vi "Database.GetProductComponentTable2.vi"(7 "ConnectionString":string, 10 "Component_SerialNo":string, 11 "Component_WabcoNo":string) -> (1 "Prod found":bool)   [LabVIEW 2016]
uses:
  <vilib>/addons/database/NI_Database_API.lvlib
  <vilib>/addons/database/_DB Variant To Data/Database Variant To Data.xnode
  <vilib>/addons/database/Connection.llb/DB Tools Open Connec (String).vi
  <vilib>/addons/database/Recordset.llb/Rec Fetch Recordset Data (R).vi
  <vilib>/addons/database/Connection.llb/Conn Execute.vi
  Controls/ProdaNG.ProductComponent.ctl
  <vilib>/addons/database/Recordset.llb/Rec Destroy - Connection.vi
panel:
  out "ProdComponents":T1[](array[typedef])
  out "error out":errorcluster
  in  "error in (no error)":errorcluster
  in  "Data":i32(listbox)
  out "sql statement":string
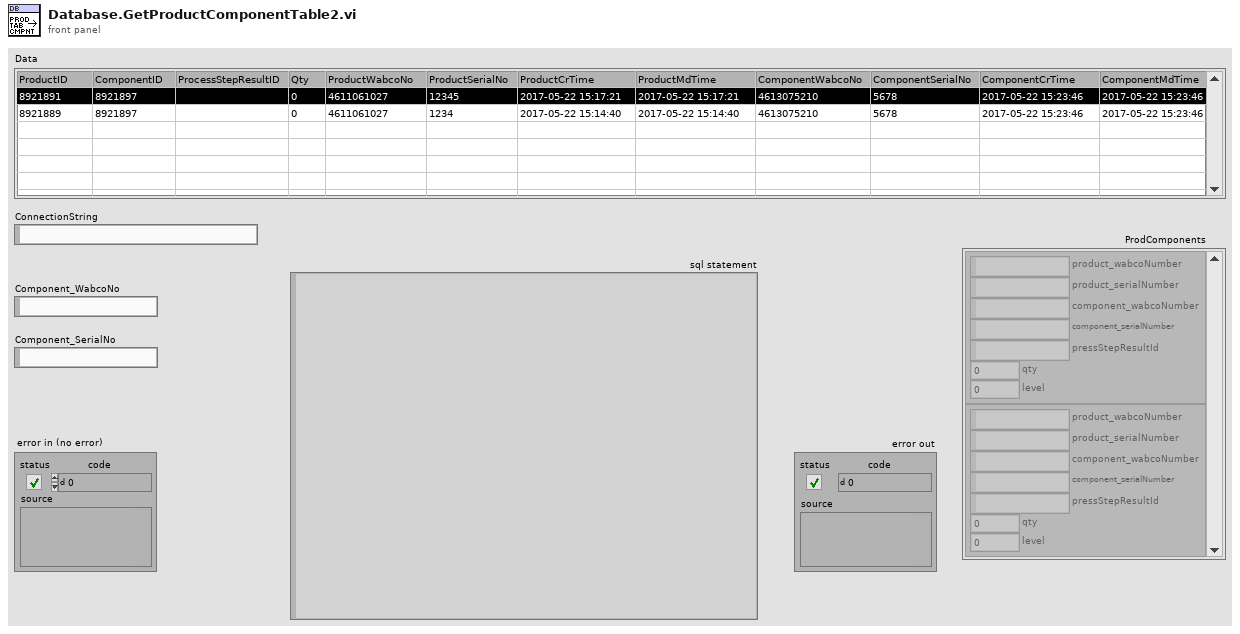
[diagram p1: front panel]
types:
  T1 = typedef "ProdaNG.ProductComponent.ctl" = cluster{"product_wabcoNumber":string, "product_serialNumber":string, "component_wabcoNumber":string, "component_serialNumber":string, "pressStepResultId":string, "qty":i32, "level":i32}
  T2 = typedef "NI_Database_API.lvlib/Conn ObjectReference.ctl" = refnum<k1>
  T3 = typedef "NI_Database_API.lvlib/Rec ObjectReference.ctl" = refnum<k1>
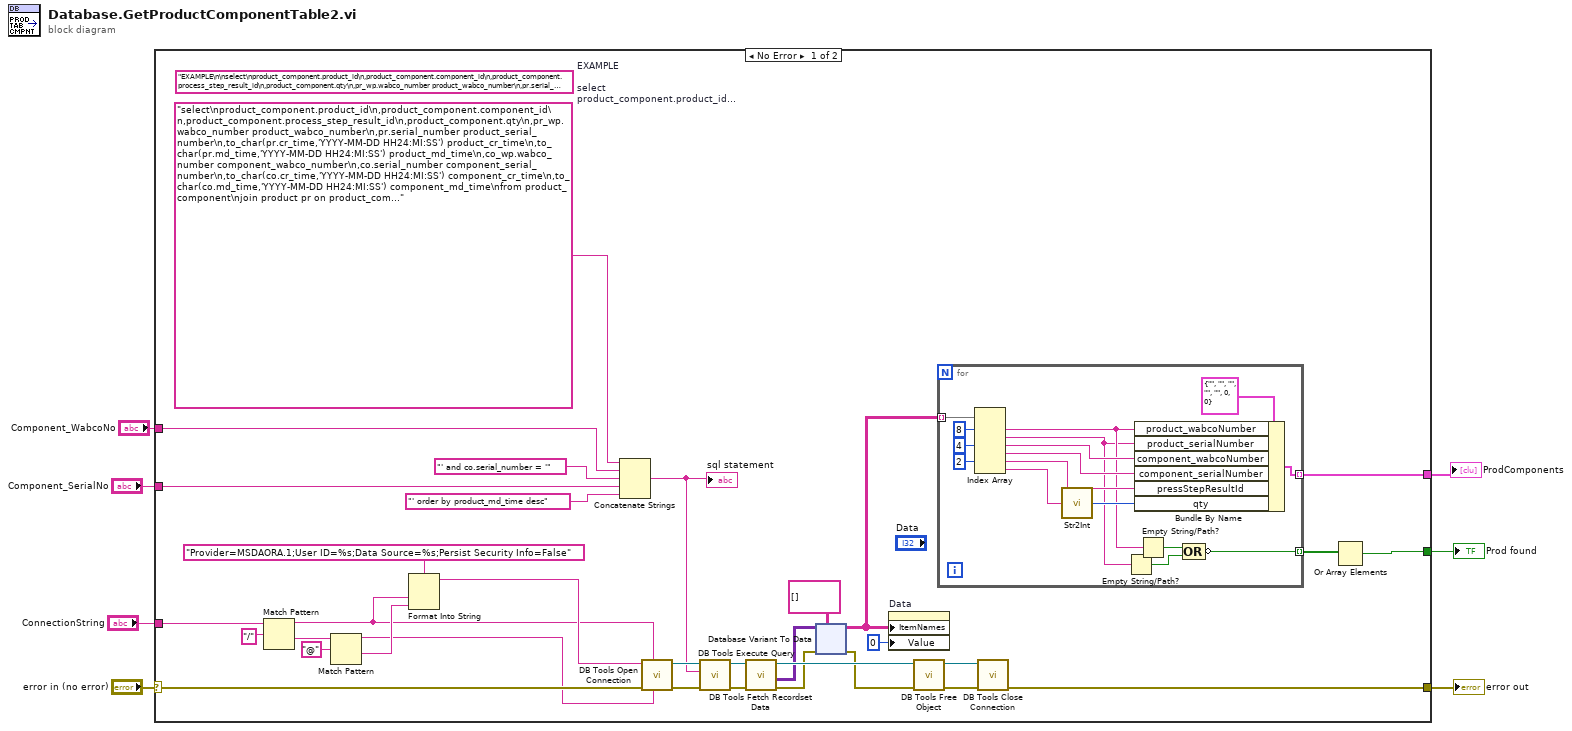
[diagram p0: block diagram]
diagram:
  n1 = case shown="No Error" "error in (no error)" {
    selector: "error in (no error)" -> [w23 w101]
    tunnel: "Component_SerialNo" -> [w26 _]
    tunnel: [w24 w101] -> w4
    tunnel: "Component_WabcoNo" -> [w22 _]
    tunnel: "ConnectionString" -> [w18 _]
    tunnel: [w10 _] -> w2
    tunnel: [w8 _] -> w1
    frame No Error {
      (unwired) "EXAMPLE\n\nselect\nproduct_component.product_id\n,product_component.component_id\n,product_component.process_step_result_id\n,product_component.qty\n,pr_wp.wabco_number product_wabco_number\n,pr.serial_number product_serial_number\n,to_char(pr.cr_time,'YYYY-MM-DD HH24:MI:SS') product_cr_time\n,to_char(pr.md_time,'YYYY-MM-DD HH24:MI:SS') product_md_time\n,co_wp.wabco_number component_wabco_number\n,co.serial_number component_serial_number\n,to_char(co.cr_time,'YYYY-MM-DD HH24:MI:SS') component_cr_time\n,to_char(co.md_time,'YYYY-MM-DD HH24:MI:SS') component_md_time\nfrom product_component\njoin product pr on product_component.product_id=pr.id\njoin wabcopart pr_wp on pr.wabco_part_id = pr_wp.id\njoin product co on product_component.component_id=co.id\njoin wabcopart co_wp on co.wabco_part_id = co_wp.id\nwhere \nco_wp.wabco_number = '4430203001'\nand co.serial_number = '03667'\norder by\nproduct_md_time\ndesc\n"  # EXAMPLE  select product_component.product_id ,product_component.component_id ,product_component.process_step_result_id ,product_component.qty ,pr_wp.wabco_number product_wabco_number ,pr.serial_number product_serial_number ,to_char(pr.cr_time,'YYYY-MM-DD HH24:MI:SS') product_cr_time ,to_char(pr.md_time,'YYYY-MM-DD HH24:MI:SS') product_md_time ,co_wp.wabco_number component_wabco_number ,co.serial_number component_serial_number ,to_char(co.cr_time,'YYYY-MM-DD HH24:MI:SS') component_cr_time ,to_char(co.md_time,'YYYY-MM-DD HH24:MI:SS') component_md_time from product_component join product pr on product_component.product_id=pr.id join wabcopart pr_wp on pr.wabco_part_id = pr_wp.id join product co on product_component.component_id=co.id join wabcopart co_wp on co.wabco_part_id = co_wp.id where  co_wp.wabco_number = '4430203001' and co.serial_number = '03667' order by product_md_time desc
      n2 = Match Pattern(string=w18, regular expression="/") -> (before substring=w14:string, after substring=w21:string)  [unwired: 1 in, 2 out]
      n3 = Match Pattern(string=w21, regular expression="@") -> (before substring=w13:string, after substring=w15:string)  [unwired: 1 in, 2 out]
      n4 = Format Into String(format string="Provider=MSDAORA.1;User ID=%s;Data Source=%s;Persist Security Info=False", w14, w15) -> (resulting string=w16:string)  [unwired: 2 in, 1 out]
      n5 = Concatenate Strings("select\nproduct_component.product_id\n,product_component.component_id\n,product_component.process_step_result_id\n,product_component.qty\n,pr_wp.wabco_number product_wabco_number\n,pr.serial_number product_serial_number\n,to_char(pr.cr_time,'YYYY-MM-DD HH24:MI:SS') product_cr_time\n,to_char(pr.md_time,'YYYY-MM-DD HH24:MI:SS') product_md_time\n,co_wp.wabco_number component_wabco_number\n,co.serial_number component_serial_number\n,to_char(co.cr_time,'YYYY-MM-DD HH24:MI:SS') component_cr_time\n,to_char(co.md_time,'YYYY-MM-DD HH24:MI:SS') component_md_time\nfrom product_component\njoin product pr on product_component.product_id=pr.id\njoin wabcopart pr_wp on pr.wabco_part_id = pr_wp.id\njoin product co on product_component.component_id=co.id\njoin wabcopart co_wp on co.wabco_part_id = co_wp.id\nwhere \nco_wp.wabco_number = '", w22, "' and co.serial_number = '", w26, "' order by product_md_time desc") -> (w28:string)
      "sql statement" <- w28
      n6 = call-poly <vilib>:"DB Tools Open Connection.vi"("password"=w13, "userID"=w14, "error in (no error)"=w23, "connection information"=w16) -> ("error out"=w39:errorcluster, "connection reference"=w36:T2)  [unwired: 4 in]
      n7 = call-poly <vilib>:"DB Tools Execute Query.vi"("error in (no error)"=w39, "SQL query"=w28, "connection reference"=w36) -> ("error out"=w40:errorcluster, "recordset reference"=w37:T3)  [unwired: 5 in]
      n8 = call-poly <vilib>:"DB Tools Fetch Recordset Data.vi"("error in (no error)"=w40, "recordset reference"=w37) -> ("error out"=w31:errorcluster, "recordset data"=w33:variant[][], "recordset reference out"=w35:T3)  [unwired: 3 in]
      n9 = xnode "Database Variant To Data"("database variant"=w33, "error in (no error)"=w31, "type"=string[][] [] ("Array")) -> ("data"=w11:string[][], "error out"=w30:errorcluster)
      n10 = property on="Data" class="MCListbox (strict)"("ItemNames"=w11, "Value"=0 ("Data")) -> ()  [unwired: 2 in, 2 out]
      n11 = call-poly <vilib>:"DB Tools Free Object.vi"("error in (no error)"=w30, "recordset reference"=w35) -> ("error out"=w38:errorcluster, "connection reference"=w34:T2)  [unwired: 8 in]
      n12 = for {
        tunnel: w11 -> [w55] mode=indexing
        tunnel: [w49] -> w10 mode=indexing
        tunnel: [w44] -> w9 mode=indexing
        n13 = Index Array(array=w55, index #1=8 ("index"), index #3=4 ("index"), index #5=2 ("index")) -> (element #1=w48:string, element #2=w47:string, element #3=w54:string, element #4=w53:string, element #5=w51:string, element #6=w50:string)  [unwired: 3 in]
        n14 = call "Str2Int.vi"("string"=w50) -> ("Numeric"=w52:i32)
        n15 = Empty String/Path?(string/path=w47) -> (empty?=w45:bool)
        n16 = Bundle By Name(cluster=T1 {"product_wabcoNumber"="", "product_serialNumber"="", "component_wabcoNumber"="", "component_serialNumber"="", "pressStepResultId"="", "qty"=0, "level"=0} ("Product_Component"), "product_wabcoNumber"=w48, "product_serialNumber"=w47, "component_wabcoNumber"=w54, "component_serialNumber"=w53, "pressStepResultId"=w51, "qty"=w52) -> (w49:T1)
        n17 = Empty String/Path?(string/path=w48) -> (empty?=w46:bool)
        n18 = Compound Arithmetic op=OR(w46, w45) -> (invert w44:bool)
      }
      n19 = call <vilib>:"DB Tools Close Connection.vi"("error in (no error)"=w38, "connection reference"=w34) -> ("error out"=w24:errorcluster)  [unwired: 5 in]
      n20 = Or Array Elements(Boolean array=w9) -> (logical OR=w8:bool)
    }
    frame Error {
    }
  }
  "Prod found" <- w1
  "error out" <- w4
  "ProdComponents" <- w2
